vi "2Dto2DSearch.vi"(10 "Array 2":u64[](array[numeric]), 11 "Array 1":u64[](array[numeric])) -> (3 "Matching numbers":dbl[](array[numeric]) format="%#_1g")   [LabVIEW 2023]
panel:
  # "Търси съвпадение на всеки елемент от вторият масив в първият.\nАко има такива ги добавя в нов масив. Индексите на елементите\nследват хронологията на откриването им."
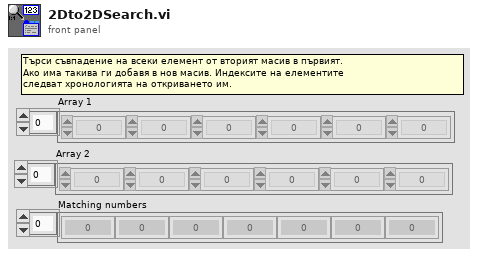
[diagram p1: front panel]
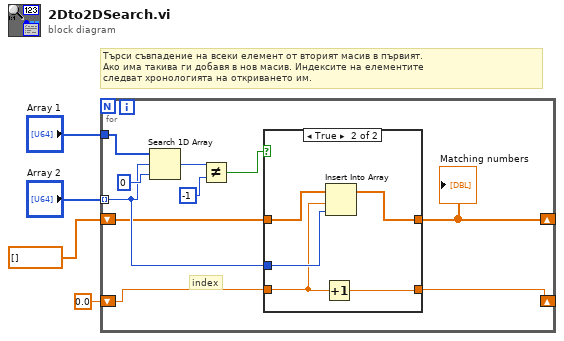
[diagram p0: block diagram]
diagram:
  # "Търси съвпадение на всеки елемент от вторият масив в първият.\nАко има такива ги добавя в нов масив. Индексите на елементите\nследват хронологията на откриването им."
  n1 = for {
    tunnel: "Array 1" -> [w14]
    tunnel: "Array 2" -> [w10] mode=indexing
    shift-right: [w9] -> _
    shift-left: dbl[] [] -> [w8]
    shift-right: [w6] -> _
    shift-left: 0.0 -> [w5]
    # "index"
    n2 = Search 1D Array(1D array=w14, element=w10, start index (0)=0) -> (index of element=w7:i32)
    n3 = Not Equal?(x=w7, y=-1) -> (x != y?=w11:bool)
    n4 = case shown="True" w11 {
      tunnel: w10 -> [_ w21]
      tunnel: w5 -> [w15 w18]
      tunnel: [w16 w20] -> w9
      tunnel: w8 -> [w16 w19]
      tunnel: [w15 w17] -> w6
      frame False {
      }
      frame True {
        n5 = Increment(x=w18) -> (x+1=w17:dbl)
        n6 = Insert Into Array "Insert Into Array"(array=w19, index=w18, new element=w21) -> (w20:dbl[])
      }
    }
    "Matching numbers" <- w9
  }
